vi "FTW-Connector-Ask.vi"(0 "FTW Actor Connector":refnum<data-value>, 5 "Request":string, 7 "Receive Timeout":i32=100 format="%dmsec", 9 "Send Timeout":i32 format="%dmsec", 11 "error in":errorcluster) -> (4 "FTW Actor Connector out":refnum<data-value>, 6 "Response":string, 8 "Roundtrip Time":dbl format="%.4psec", 15 "error out":errorcluster)   [LabVIEW 2014]
uses:
  core/FTW-Connector-Core-Type.ctl
  error/FTW-ERR-ThrowGenericError.vi
  error/FTW-ERR-ThrowError.vi
  error/FTW-ERR-NoErrorConstant.vi
  error/FTW-ERR-CallChain.vi
  string/FTW-STR-ReplaceWhitespace.vi
panel:
  # "Inputs"
  # "Outputs"
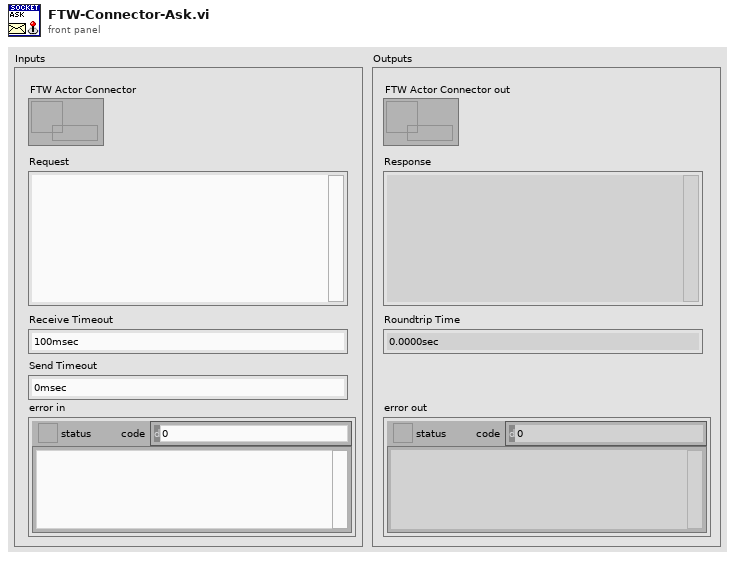
[diagram p1: front panel]
types:
  T1 = typedef "FTW-Connector-Core-Type.ctl" = cluster{"Socket":i64}
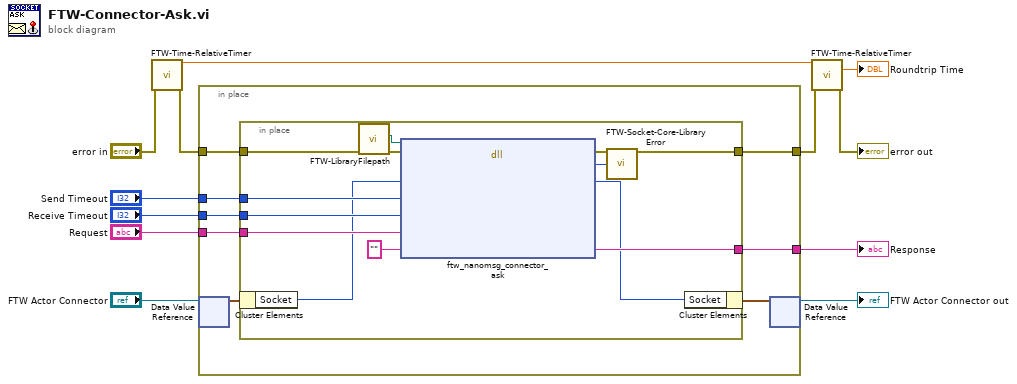
[diagram p0: block diagram]
diagram:
  n1 = call "FTW-Time-RelativeTimer.vi"("error in"="error in") -> ("Current Time"=w3:dbl, "error out"=w5:errorcluster)  [unwired: 12 in, 1 out]
  n2 = in-place {
    in-place-border: w5 -> [w20]
    in-place-border: [w19] -> w4
    in-place-border: [w18] -> w8
    in-place-border: "Send Timeout" -> [w17]
    in-place-border: "Receive Timeout" -> [w16]
    in-place-border: "Request" -> [w15]
    n3 = in-place-dvr #1("FTW Actor Connector") -> (w14:T1)  [unwired: 1 out]
    n4 = in-place {
      in-place-border: w20 -> [w33]
      in-place-border: [w31] -> w19
      in-place-border: [w30] -> w18
      in-place-border: w17 -> [w27]
      in-place-border: w16 -> [w26]
      in-place-border: w15 -> [w24]
      n5 = in-place-cluster #2(w14) -> ("Socket"=w22:i64)
      n6 = call "FTW-LibraryFilepath.vi"("error in"=w33) -> ("error out"=w28:errorcluster, "Library Filepath"=w29:path)  [unwired: 8 in, 1 out]
      n7 = dll-call lib="?" fn="ftw_nanomsg_connector_ask"(path in=w29, error in=w28, "Socket Handle"=w22, "Send Timeout"=w27, "Recv Timeout"=w26, "Request"=w24, "Response"="") -> (error out=w32:errorcluster, "Return Value"=w25:i64, "Socket Handle"=w21:i64, "Response"=w30:string)  [unwired: 4 in, 1 out]
      n8 = call "FTW-Socket-Core-LibraryError.vi"("error in"=w32, "Return Value"=w25) -> ("error out"=w31:errorcluster)  [unwired: 13 in]
      n9 = in-place-cluster #2("Socket"=w21) -> (w13:T1)
    }
    n10 = in-place-dvr #1(w13) -> (→"FTW Actor Connector out":refnum<data-value>)  [unwired: 1 out]
  }
  "Response" <- w8
  n11 = call "FTW-Time-RelativeTimer.vi"("Previous Time"=w3, "error in"=w4) -> ("Elapsed Time"=→"Roundtrip Time":dbl, "error out"=→"error out":errorcluster)  [unwired: 11 in, 1 out]
